vi "_TangoDeviceCommandsInfo.vi"(2 "error in":errorcluster, 3 "device name":string) -> (0 "error out":errorcluster, 1 "commands_info":T1[](array[typedef]))   [LabVIEW 2014, in "tango.lvlib"]
uses:
  tango.lvlib
  Common VIs/Typedefs/_CommandInfo_t.ctl
  tango_binding.dll
panel:
  # "CommandInfo.level\n-----------------------\n\tOPERATOR = 0\n EXPERT = 1"
  # "CommandInfo.in-out-type\n-----------------------\n\tDEV_VOID = 0\n\tDEV_BOOLEAN = 1\n\tDEV_SHORT = 2\n\tDEV_LONG = 3\n\tDEV_FLOAT = 4\n\tDEV_DOUBLE = 5\n\tDEV_USHORT = 6\n\tDEV_ULONG = 7\n\tDEV_STRING = 8\n\tDEVVAR_CHARARRAY = 9\n\tDEVVAR_SHORTARRAY = 10\n\tDEVVAR_LONGARRAY = 11\n\tDEVVAR_FLOATARRAY = 12\n\tDEVVAR_DOUBLEARRAY = 13\n\tDEVVAR_USHORTARRAY = 14\n\tDEVVAR_ULONGARRAY = 15\n\tDEVVAR_STRINGARRAY = 16\n\tDEVVAR_LONGSTRINGARRAY = 17\n\tDEVVAR_DOUBLESTRINGARRAY = 18\n\tDEV_STATE = 19\n\tCONST_DEV_STRING = 20\n\tDEVVAR_BOOLEANARRAY = 21\n\tDEV_UCHAR = 22\n\tDEV_LONG64 = 23\n\tDEV_ULONG64 = 24\n\tDEVVAR_LONG64ARRAY = 25\n\tDEVVAR_ULONG64ARRAY = 26\n\tDEV_INT = 27\n\tDEV_ENCODED = 28"
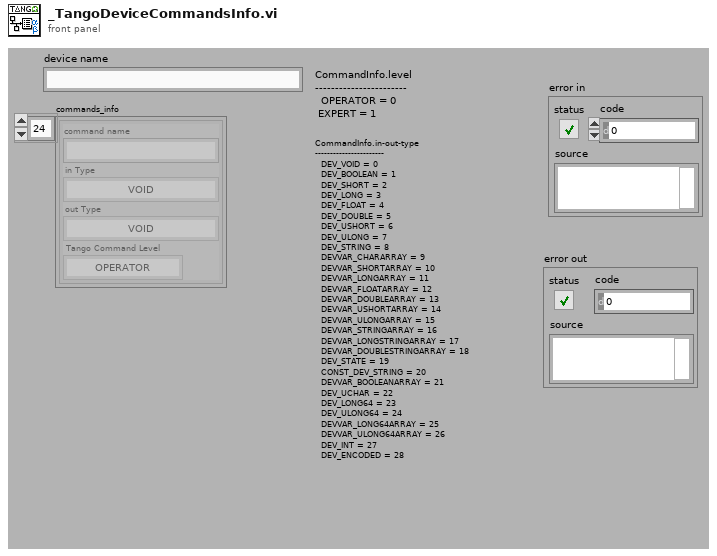
[diagram p1: front panel]
types:
  T1 = typedef "tango.lvlib/_CommandInfo_t.ctl" = cluster{"command name":string, "in Type":enum16{"VOID", "BOOLEAN", "SHORT", "LONG", "FLOAT", "DOUBLE", "USHORT", "ULONG", "STRING", "CHAR_ARRAY", "SHORT_ARRAY", "LONG_ARRAY", "FLOAT_ARRAY", "DOUBLE_ARRAY", "USHORT_ARRAY", "ULONG_ARRAY", "STRING_ARRAY", "LONG_STRING_ARRAY", "DOUBLE_STRING_ARRAY", "STATE", "CONST_STRING", "BOOLEAN_ARRAY", "UCHAR", "LONG64", "ULONG64", "LONG64_ARRAY", "ULONG64_ARRAY", "INT (not supported)", "ENCODED (not supported)", "ENUM", "PIPE_BLOB (not supported)", "STATE_ARRAY", "UNKNOW_DATA_TYPE"}, "out Type":enum16{"VOID", "BOOLEAN", "SHORT", "LONG", "FLOAT", "DOUBLE", "USHORT", "ULONG", "STRING", "CHAR_ARRAY", "SHORT_ARRAY", "LONG_ARRAY", "FLOAT_ARRAY", "DOUBLE_ARRAY", "USHORT_ARRAY", "ULONG_ARRAY", "STRING_ARRAY", "LONG_STRING_ARRAY", "DOUBLE_STRING_ARRAY", "STATE", "CONST_STRING", "BOOLEAN_ARRAY", "UCHAR", "LONG64", "ULONG64", "LONG64_ARRAY", "ULONG64_ARRAY", "INT (not supported)", "ENCODED (not supported)", "ENUM", "PIPE_BLOB (not supported)", "STATE_ARRAY", "UNKNOW_DATA_TYPE"}, "Tango Command Level":enum16{"OPERATOR", "EXPERT", "UNKNOWN_LEVEL"}}
  T2 = cluster{"command name":string, "in type":i16, "out type":i16, "level":i16}[]
  T3 = cluster{"command name":string, "in type":i16, "out type":i16, "level":i16}
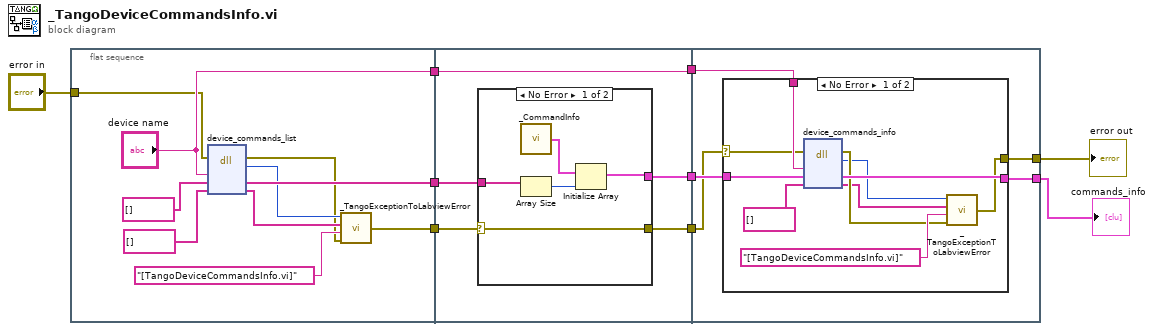
[diagram p0: block diagram]
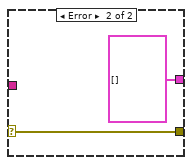
[diagram p2: hidden frame]
diagram:
  n1 = flat-sequence {
    tunnel: [w17] -> w9
    tunnel: ["device name"] -> w8
    tunnel: [w12] -> w5
    tunnel: "error in" -> [w10]
    tunnel: w9 -> [w21]
    tunnel: [w24] -> w7
    tunnel: [w23] -> w6
    tunnel: w8 -> [w23]
    tunnel: w5 -> [w22]
    tunnel: [w20] -> w4
    tunnel: w7 -> [w36]
    tunnel: w6 -> [w35]
    tunnel: w4 -> [w34]
    tunnel: [w33] -> w3
    tunnel: [w32] -> w2
    frame #0 {
      n2 = dll-call lib="tango_binding.*" fn="device_commands_list"(error in=w10, "dev_name"="device name", "attributes_list"=string[] [] ("Error Stack"), "error_stack"=string[] [] ("Error Stack")) -> (error out=w11:errorcluster, "return type"=w13:i32, "attributes_list"=w17:string[], "error_stack"=w14:string[])  [unwired: 3 in, 1 out]
      n3 = call "_TangoExceptionToLabviewError.vi"("error in"=w11, "location"="[TangoDeviceCommandsInfo.vi]", "error stack"=w14, "error code"=w13) -> ("error out"=w12:errorcluster)
    }
    frame #1 {
      n4 = case shown="No Error" w22 {
        selector: w22 -> [w25 w30]
        tunnel: [w27 T2 []] -> w24
        tunnel: w21 -> [w26 _]
        tunnel: [w25 w30] -> w20
        frame No Error {
          n5 = call "_CommandInfo.vi"() -> ("command info"=w28:T3)
          n6 = Array Size(array=w26) -> (size(s)=w29:i32)
          n7 = Initialize Array(w28, w29) -> (w27:T2)
        }
        frame Error {
        }
      }
    }
    frame #2 {
      n8 = case shown="No Error" w34 {
        selector: w34 -> [w41 w48]
        tunnel: w36 -> [w45 w47]
        tunnel: w35 -> [w44 _]
        tunnel: [w37 w48] -> w33
        tunnel: [w43 w47] -> w32
        frame No Error {
          n9 = dll-call lib="tango_binding.*" fn="device_commands_info"(error in=w41, "dev_name"=w44, "commands_info"=w45, "error_stack"=string[] [] ("Error Stack")) -> (error out=w40:errorcluster, "return type"=w39:i32, "commands_info"=w43:T2, "error_stack"=w38:string[])  [unwired: 3 in, 1 out]
          n10 = call "_TangoExceptionToLabviewError.vi"("error in"=w40, "location"="[TangoDeviceCommandsInfo.vi]", "error stack"=w38, "error code"=w39) -> ("error out"=w37:errorcluster)
        }
        frame Error {
        }
      }
    }
  }
  "error out" <- w3
  "commands_info" <- w2
